vi "Edgertronic-:download copy.vi"(5 "Setup":T2={"URL"="130.64.16.195", "remote port"=80, "mode (standard)"=enum."Standard"}) -> (0 "error out":errorcluster, 1 "Download":T1={"Download file extension"="20140911165611", "Connection Information:"=""}, 2 "data out":string="HTTP/1.0 200 OK\r\nContent-Type: text/html; charset=utf-8\r\nContent-Length: 313\r\nConnection: close\r\nDate: Tue, 16 Jun 2015 13:54:12 GMT\r\nServer: lighttpd/1.4.11 (edgertonic slow motion camera)\r\n\r\n{\"build_date\": \"20150112\", \"sw_build_date\": \"20140911165611\", \"fpga_initialized\": 1, \"hardware_revision\": 6, \"model_number\": 1, \"home_dir\": \"/home/root/ss-web\", \"ir_filter\": 1, \"mac_addr\": \"00:1B:C5:09:61:4D\", \"serial_console_enabled\": false, \"serial_number\": 333, \"fpga_version\": 70, \"hardware_configuration\": 1}")   [LabVIEW 2012]
doc: "This VI downloads the last saved video marking data with MIME type video/quicktime."
panel:
  in  "GET Cmd":string="/download"
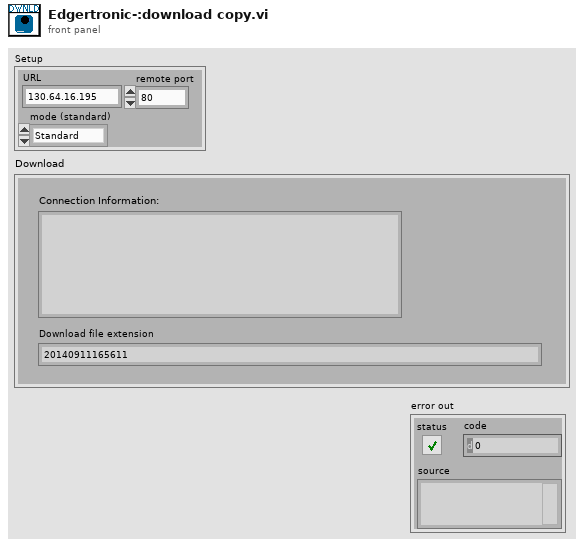
[diagram p1: front panel]
types:
  T1 = cluster{"Download file extension":string, "Connection Information:":string}
  T2 = cluster{"URL":string, "remote port":u16, "mode (standard)":enum16{"Standard", "Buffered", "CRLF", "Immediate"}}
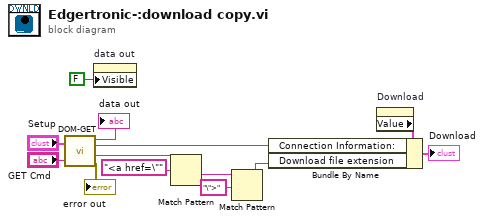
[diagram p0: block diagram]
diagram:
  n1 = call <userlib>:"DOM-GET.vi"("Setup"="Setup", "GET Command"="GET Cmd") -> ("Data Out from Camera"=→"data out":string, "Connection Information"=w4:string, "Value String"=w3:string, "error out"=→"error out":errorcluster)
  n2 = property on="data out" class="Str"("Visible"=FALSE) -> ()  [unwired: 2 in, 2 out]
  n3 = Match Pattern(string=w3, regular expression="<a href=\"") -> (after substring=w8:string)  [unwired: 1 in, 3 out]
  n4 = Match Pattern(string=w8, regular expression="\">") -> (before substring=w5:string)  [unwired: 1 in, 3 out]
  n5 = property on="Download" class="Clust (strict)"() -> ("Value"=w2:T1)  [unwired: 2 in, 2 out]
  n6 = Bundle By Name(cluster=w2, "Connection Information:"=w4, "Download file extension"=w5) -> (→"Download":T1)
